vi "InitRef.vi"(8 "error in (no error)":errorcluster, 10 "Ref":T1, 11 "Caller in":refnum<class "Caller.lvclass">) -> (0 "error out":errorcluster, 3 "Caller out":refnum<class "Caller.lvclass">)   [LabVIEW 2020, in "Caller.lvlib" / "Caller.lvclass"]
uses:
  Caller.lvclass
  _ctrl/ctrl_ref.ctl
  Caller.lvclass/Caller.ctl
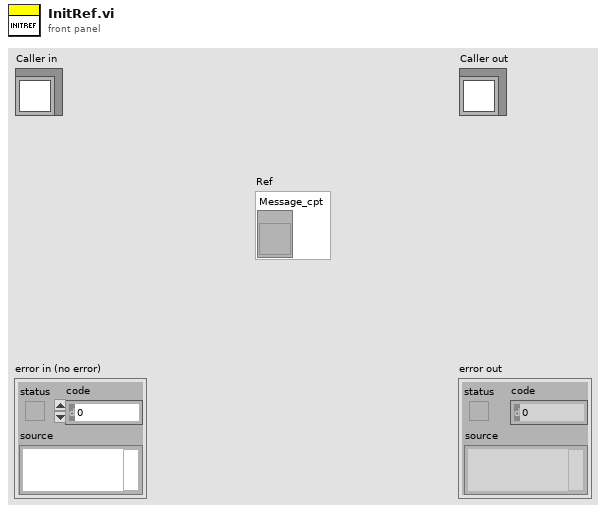
[diagram p1: front panel]
types:
  T1 = typedef "ctrl_ref.ctl" = cluster{"Message_cpt":refnum<vi>}
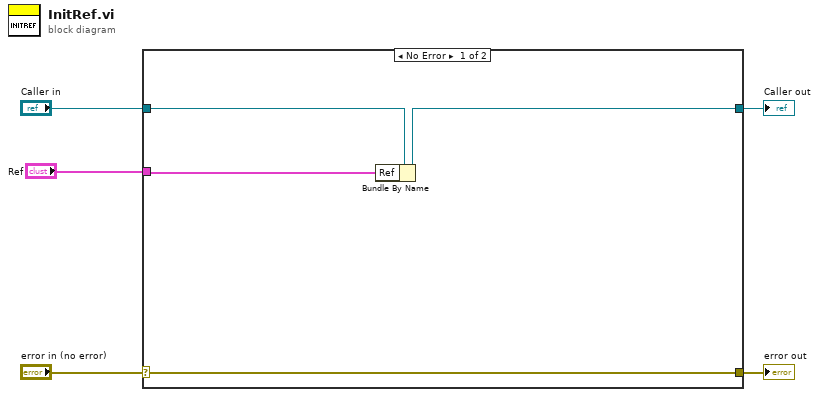
[diagram p0: block diagram]
diagram:
  n1 = case shown="No Error" "error in (no error)" {
    selector: "error in (no error)" -> [w8 w11]
    tunnel: [w8 w11] -> w4
    tunnel: [w7 w10] -> w2
    tunnel: "Caller in" -> [w9 w10]
    tunnel: "Ref" -> [w6 _]
    frame No Error {
      n2 = Bundle By Name(cluster=w9, "Ref"=w6) -> (w7:refnum<class "Caller.lvclass">)
    }
    frame Error {
    }
  }
  "error out" <- w4
  "Caller out" <- w2
